vi "iXon_Shutdown.vi"(8 "error in (no error)":errorcluster, 11 "TurnOFFCooler":bool=TRUE caption="PD Correction") -> (0 "error out":errorcluster, 3 "Current Temp":i32)   [LabVIEW 2018]
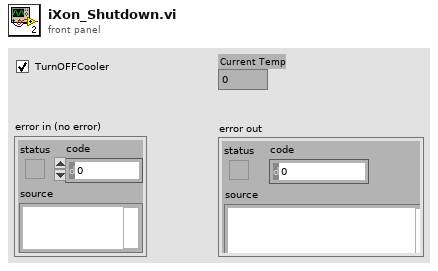
[diagram p1: front panel]
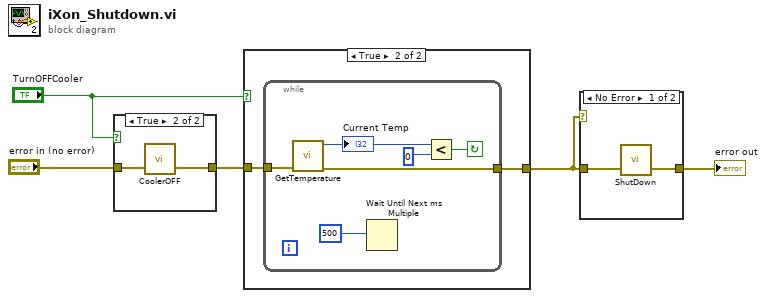
[diagram p0: block diagram]
diagram:
  n1 = case shown="True" "TurnOFFCooler" {
    tunnel: "error in (no error)" -> [w6 w8]
    tunnel: [w6 w7] -> w3
    frame False {
    }
    frame True {
      n2 = call <userlib>:"CoolerOFF.vi"("error in (no error)"=w8) -> ("error out"=w7:errorcluster)  [unwired: 1 in, 1 out]
    }
  }
  n3 = case shown="True" "TurnOFFCooler" {
    tunnel: w3 -> [w9 w11]
    tunnel: [w9 w10] -> w1
    frame False {
    }
    frame True {
      n4 = while {
        tunnel: w11 -> [w13]
        tunnel: [w12] -> w10
        stop <- w16 continue-if-true
        n5 = call <userlib>:"GetTemperature.vi"("error in (no error)"=w13) -> ("error out"=w12:errorcluster, "temperature"=w15:i32)  [unwired: 3 in, 2 out]
        "Current Temp" <- w15
        n6 = Wait Until Next ms Multiple(millisecond multiple=u32 500) -> ()  [unwired: 1 out]
        n7 = Less?(x=w15, y=i16 0) -> (x < y?=w16:bool)
      }
    }
  }
  n8 = case shown="No Error" w1 {
    tunnel: w1 -> [w19 w20]
    tunnel: [w18 w20] -> w2
    frame No Error {
      n9 = call <userlib>:"ShutDown.vi"("error in (no error)"=w19) -> ("error out"=w18:errorcluster)  [unwired: 1 in, 1 out]
    }
    frame Error {
    }
  }
  "error out" <- w2
